vi "Open.vi"(7 "Port (80)":u16=80, 8 "Error In":errorcluster, 9 "Password":string="password", 10 "Username":string="samk", 11 "Hostname / IP":string="localhost") -> (0 "Error Out":errorcluster, 3 "XBMC Ref":T1)   [LabVIEW 2013, in "LVH-XBMC.lvlib"]
uses:
  LVH-XBMC.lvlib
  Private/Type Defs/XBMC Ref.ctl
  <vilib>/httpClient/ClientHandle.ctl
  Private/Type Defs/Input.Action.ctl
  Private/Type Defs/ID FGV State.ctl
  <vilib>/httpClient/LabVIEWHTTPClient.lvlib
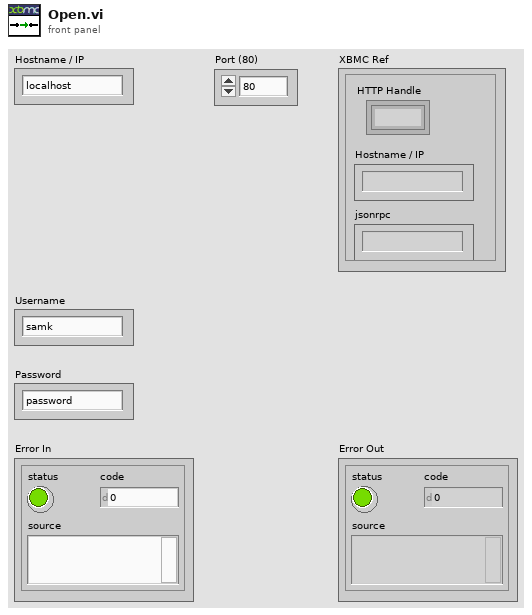
[diagram p1: front panel]
types:
  T1 = typedef "LVH-XBMC.lvlib/XBMC Ref.ctl" = cluster{"HTTP Handle":T2, "Hostname / IP":string, "jsonrpc":string}
  T2 = typedef "LabVIEWHTTPClient.lvlib/ClientHandle.ctl" = refnum<k1>
  T3 = typedef "LVH-XBMC.lvlib/Input.Action.ctl" = enum16{"left", "right", "up", "down", "pageup", "pagedown", "select", "highlight", "parentdir", "parentfolder", "back", "previousmenu", "info", "pause", "stop", "skipnext", "skipprevious", "fullscreen", "aspectratio", "stepforward", "stepback", "bigstepforward", "bigstepback", "chapterorbigstepforward", "chapterorbigstepback", "osd", "showsubtitles", "nextsubtitle", "codecinfo", "nextpicture", "previouspicture", "zoomout", "zoomin", "playlist", "queue", "zoomnormal", "zoomlevel1", "zoomlevel2", "zoomlevel3", "zoomlevel4", "zoomlevel5", "zoomlevel6", "zoomlevel7", "zoomlevel8", "zoomlevel9", "nextcalibration", "resetcalibration", "analogmove", "rotate", "rotateccw", "close", "subtitledelayminus", "subtitledelay", "subtitledelayplus", "audiodelayminus", "audiodelay", "audiodelayplus", "subtitleshiftup", "subtitleshiftdown", "subtitlealign", "audionextlanguage", "verticalshiftup", "verticalshiftdown", "nextresolution", "audiotoggledigital", "number0", "number1", "number2", "number3", "number4", "number5", "number6", "number7", "number8", "number9", "osdleft", "osdright", "osdup", "osddown", "osdselect", "osdvalueplus", "osdvalueminus", "smallstepback", "fastforward", "rewind", "play", "playpause", "switchplayer", "delete", "copy", "move", "mplayerosd", "hidesubmenu", "screenshot", "rename", "togglewatched", "scanitem", "reloadkeymaps", "volumeup", "volumedown", "mute", "backspace", "scrollup", "scrolldown", "analogfastforward", "analogrewind", "moveitemup", "moveitemdown", "contextmenu", "shift", "symbols", "cursorleft", "cursorright", "showtime", "analogseekforward", "analogseekback", "showpreset", "presetlist", "nextpreset", "previouspreset", "lockpreset", "randompreset", "increasevisrating", "decreasevisrating", "showvideomenu", "enter", "increaserating", "decreaserating", "togglefullscreen", "nextscene", "previousscene", "nextletter", "prevletter", "jumpsms2", "jumpsms3", "jumpsms4", "jumpsms5", "jumpsms6", "jumpsms7", "jumpsms8", "jumpsms9", "filter", "filterclear", "filtersms2", "filtersms3", "filtersms4", "filtersms5", "filtersms6", "filtersms7", "filtersms8", "filtersms9", "firstpage", "lastpage", "guiprofile", "red", "green", "yellow", "blue", "increasepar", "decreasepar", "volampup", "volampdown", "createbookmark", "createepisodebookmark", "settingsreset", "settingslevelchange", "stereomode", "nextstereomode", "previousstereomode", "togglestereomode", "stereomodetomono", "channelup", "channeldown", "previouschannelgroup", "nextchannelgroup", "playpvr", "playpvrtv", "playpvrradio", "record", "leftclick", "rightclick", "middleclick", "doubleclick", "wheelup", "wheeldown", "mousedrag", "mousemove", "tap", "longpress", "pangesture", "zoomgesture", "rotategesture", "swipeleft", "swiperight", "swipeup", "swipedown", "noop"}
  T4 = typedef "LVH-XBMC.lvlib/ID FGV State.ctl" = enum16{"Init", "Peek", "Get++"}
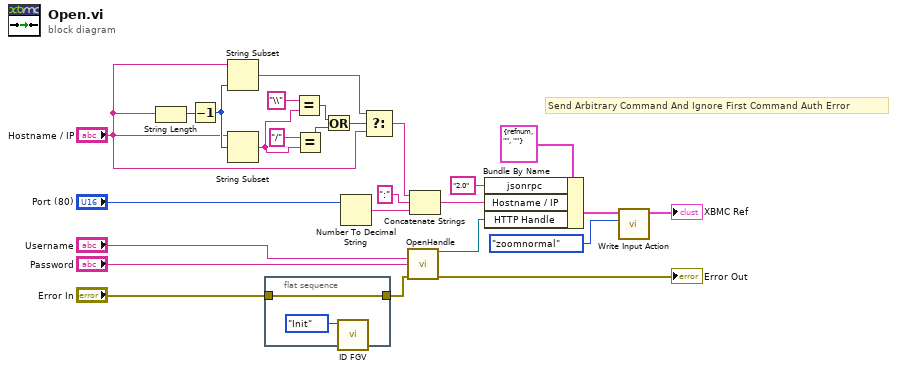
[diagram p0: block diagram]
diagram:
  # "Send Arbitrary Command And Ignore First Command Auth Error"
  n1 = String Length(string="Hostname / IP") -> (length=w12:i32)
  n2 = Decrement(x=w12) -> (x-1=w5:i32)
  n3 = String Subset(string="Hostname / IP", length (rest)=w5) -> (substring=w4:string)  [unwired: 1 in]
  n4 = String Subset(string="Hostname / IP", offset (0)=w5) -> (substring=w6:string)  [unwired: 1 in]
  n5 = flat-sequence {
    tunnel: [w27] -> w16
    tunnel: "Error In" -> [w27]
    frame #0 {
      n6 = call "ID FGV.vi"("FGV State"=ID_FGV_State."Init") -> ()  [unwired: 10 in, 1 out]
    }
  }
  n7 = Equal?(x="\\" ("y"), y=w6) -> (x = y?=w8:bool)
  n8 = Equal?(x="/" ("y"), y=w6) -> (x = y?=w10:bool)
  n9 = Or(x=w8, y=w10) -> (x .or. y?=w7:bool)
  n10 = Number To Decimal String(number="Port (80)") -> (decimal integer string=w14:string)  [unwired: 1 in]
  n11 = Select(t=w4, s=w7, f="Hostname / IP") -> (s? t:f=w1:string)
  n12 = call <vilib>:"OpenHandle.vi"("username"="Username", "password"="Password", "error in (no error)"=w16) -> ("client handle out"=w23:T2, "error out"=→"Error Out":errorcluster)  [unwired: 11 in]
  n13 = Concatenate Strings(w1, ":" ("string"), w14) -> (w2:string)
  n14 = Bundle By Name(cluster=T1 {"HTTP Handle"=refnum, "Hostname / IP"="", "jsonrpc"=""} ("XBMC Ref"), "jsonrpc"="2.0", "Hostname / IP"=w2, "HTTP Handle"=w23) -> (w20:T1)
  n15 = call "Write Input Action.vi"("Input Action"=Input.Action."zoomnormal", "XBMC Ref"=w20) -> ("XBMC Ref"=→"XBMC Ref":T1)  [unwired: 8 in, 1 out]
